vi "主动发送数据生成Condition(子VI).vi"(8 "数据发送协议":enum16{"2005-212协议", "2017-212协议"}(ring)=enum."2017-212协议", 9 "database":string, 10 "Label.Text":string, 11 "数值":i32) -> (2 "columns":string[](array[string])=["时间", "测量模式", "数据类型", "检测值", "单位", "数据标识"], 3 "CONDITION":string)   [LabVIEW 2016, in "数据传输系统.lvlib"]
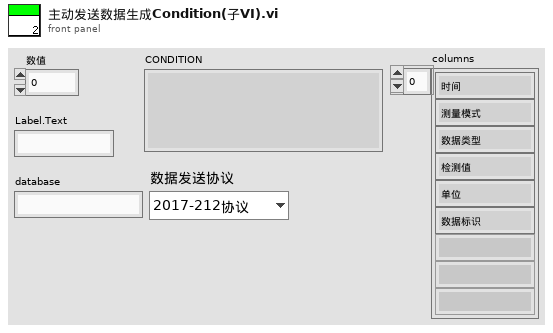
[diagram p1: front panel]
types:
  T1 = cluster{"time1":string, "time2":string, "time3":string, "time4":string, "time5":string, "time6":string, "time7":string, "time8":string, "time9":string, "time10":string, "time11":string, "time12":string, "time13":string, "time14":string, "time15":string, "time16":string, "time17":string, "time18":string, "time19":string, "time20":string, "time21":string, "time22":string, "time23":string, "time24":string, "time25":string, "time26":string, "time27":string, "time28":string, "time29":string, "time30":string, "time31":string}
  T2 = typedef "LVDateTimeRec.ctl" = cluster{"秒数的小数部分":dbl, "秒":i32, "分":i32, "时":i32, "日":i32, "月":i32, "年":i32, "天数（周）":i32, "天数（年）":i32, "DST":i32}
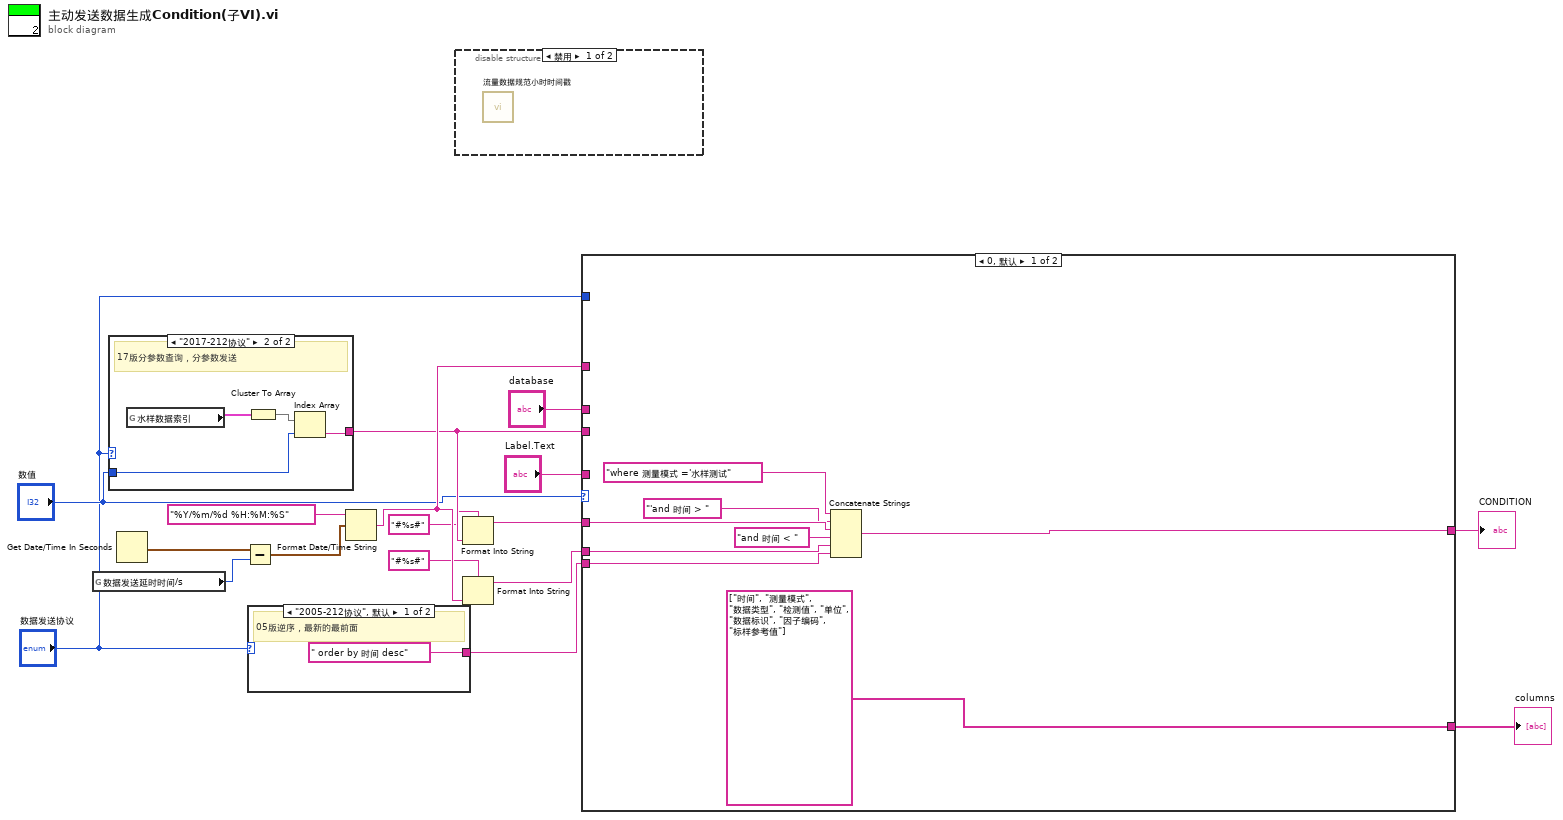
[diagram p0: block diagram]
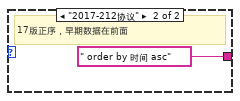
[diagram p3: hidden frame]
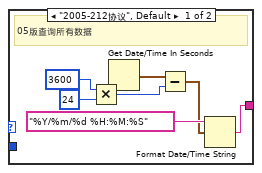
[diagram p4: hidden frame]
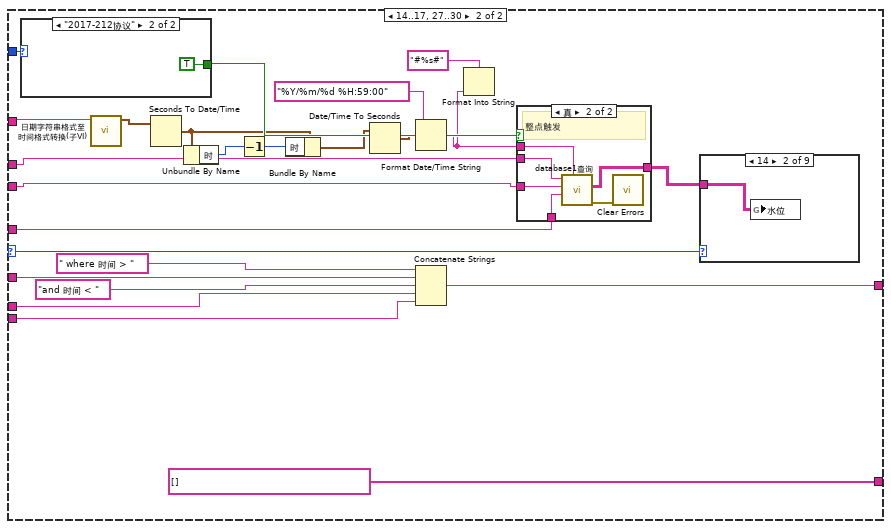
[diagram p5: hidden frame]
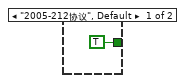
[diagram p6: hidden frame]
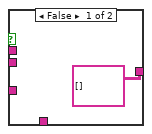
[diagram p7: hidden frame]
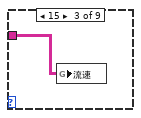
[diagram p9: hidden frame]
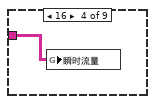
[diagram p10: hidden frame]
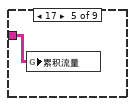
[diagram p11: hidden frame]
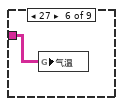
[diagram p12: hidden frame]
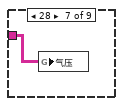
[diagram p13: hidden frame]
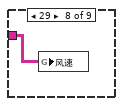
[diagram p14: hidden frame]
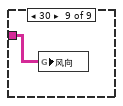
[diagram p15: hidden frame]
diagram:
  n1 = global read "断电保存全局.vi" "数据发送延时时间/s"() -> (w3:i32)
  n2 = case shown="\"2017-212协议\"" "数据发送协议" {
    tunnel: [w23 w25] -> w16
    tunnel: "数值" -> [_ w26]
    frame "2005-212协议", Default {
      # "05版查询所有数据"
      n3 = Multiply(x=3600, y=24) -> (x*y=w18:i32)
      n4 = Get Date/Time In Seconds() -> (seconds since 1Jan1904=w22:timestamp)
      n5 = Subtract(x=w22, y=w18) -> (x-y=w21:timestamp)
      n6 = Format Date/Time String(time format string (%c)="%Y/%m/%d %H:%M:%S" ("时间格式字符串(%c)"), seconds (now)=w21) -> (date/time string=w23:string)  [unwired: 1 in]
    }
    frame "2017-212协议" {
      # "17版分参数查询，分参数发送"
      n7 = global read "全局 水样时间.vi" "水样数据索引"() -> (w27:T1)
      n8 = Cluster To Array(cluster=w27) -> (array=w28:string[])
      n9 = Index Array(array=w28, index=w26) -> (element=w25:string)
    }
  }
  n10 = Get Date/Time In Seconds() -> (seconds since 1Jan1904=w2:timestamp)
  n11 = Subtract(x=w2, y=w3) -> (x-y=w1:timestamp)
  n12 = case shown="\"2005-212协议\", 默认" "数据发送协议" {
    tunnel: [" order by 时间 desc" ("字符串") " order by 时间 asc" ("字符串")] -> w6
    frame "2005-212协议", Default {
      # "05版逆序，最新的最前面"
    }
    frame "2017-212协议" {
      # "17版正序，早期数据在前面"
    }
  }
  n13 = Format Date/Time String(time format string (%c)="%Y/%m/%d %H:%M:%S" ("时间格式字符串(%c)"), seconds (now)=w1) -> (date/time string=w17:string)  [unwired: 1 in]
  n14 = disable-structure shown="禁用" {
    frame Disabled {
      n15 = call "流量数据规范小时时间戳.vi"() -> ()  [unwired: 11 in, 1 out]
    }
    frame Enabled {
    }
  }
  n16 = Format Into String(format string="#%s#" ("初始字符串"), w16) -> (resulting string=w10:string)  [unwired: 2 in, 1 out]
  n17 = Format Into String(format string="#%s#" ("初始字符串"), w17) -> (resulting string=w12:string)  [unwired: 2 in, 1 out]
  n18 = case shown="0, 默认" "数值" {
    selector: "数值" -> [_ w55]
    tunnel: w10 -> [w38 w59]
    tunnel: [w37 w60] -> w11
    tunnel: w12 -> [w35 w40]
    tunnel: "database" -> [_ w58]
    tunnel: "Label.Text" -> [_ w57]
    tunnel: w16 -> [_ w39]
    tunnel: w17 -> [_ w43]
    tunnel: w6 -> [w32 w54]
    tunnel: [string[] ["时间", "测量模式", "数据类型", "检测值", "单位", "数据标识", "因子编码", "标样参考值"] ("columns") string[] [] ("columns")] -> w5
    tunnel: "数据发送协议" -> [_ w51]
    frame 0, Default {
      n19 = Concatenate Strings("where 测量模式 ='水样测试" ("condition"), "'and 时间 > ", w38, "and 时间 < " ("字符串"), w35, w32) -> (w37:string)
    }
    frame 14..17, 27..30 {
      n20 = case shown="\"2017-212协议\"" w51 {
        tunnel: [TRUE TRUE] -> w53
        frame "2005-212协议", Default {
        }
        frame "2017-212协议" {
        }
      }
      n21 = call "日期字符串格式至时间格式转换(子VI).vi"("data[0]"=w43) -> ("time stamp"=w46:timestamp)  [unwired: 10 in]
      n22 = Seconds To Date/Time(time stamp (now)=w46) -> (date time rec=w48:T2)  [unwired: 1 in]
      n23 = Unbundle By Name(w48) -> ("时"=w49:i32)
      n24 = Decrement(x=w49) -> (x-1=w50:i32)
      n25 = Bundle By Name(cluster=w48, "时"=w50) -> (w47:T2)
      n26 = Date/Time To Seconds(2:w47) -> (0:w45:timestamp)  [unwired: 1 in]
      n27 = Format Date/Time String(time format string (%c)="%Y/%m/%d %H:59:00" ("时间格式字符串(%c)"), seconds (now)=w45) -> (date/time string=w41:string)  [unwired: 1 in]
      n28 = Concatenate Strings(" where 时间 > ", w59, "and 时间 < " ("字符串"), w40, w54) -> (w60:string)
      n29 = Format Into String(format string="#%s#" ("初始字符串"), w41) -> ()  [unwired: 2 in, 2 out]
      n30 = case shown="真" w53 {
        tunnel: w58 -> [_ w71]
        tunnel: w57 -> [_ w70]
        tunnel: [string[][] [] ("data") w69] -> w56
        tunnel: w41 -> [_ w68]
        tunnel: w39 -> [_ w66]
        frame False {
        }
        frame True {
          # "整点触发"
          n31 = call "database1查询.vi"("时间2"=w68, "table"=w70, "时间1"=w66, "database"=w71) -> ("error out"=w67:errorcluster, "data"=w69:string[][])  [unwired: 4 in, 1 out]
          n32 = call <vilib>:"Clear Errors.vi"("error in (no error)"=w67) -> ()  [unwired: 5 in, 2 out]
        }
      }
      n33 = case shown="14" w55 {
        tunnel: w56 -> [_ w72 w73 w74 w75 w76 w77 w78 w79]
        frame 0, Default {
        }
        frame 14 {
          n34 = global write "全局 所有参数.vi" "水位"(w72) -> ()
        }
        frame 15 {
          n35 = global write "全局 所有参数.vi" "流速"(w73) -> ()
        }
        frame 16 {
          n36 = global write "全局 所有参数.vi" "瞬时流量"(w74) -> ()
        }
        frame 17 {
          n37 = global write "全局 所有参数.vi" "累积流量"(w75) -> ()
        }
        frame 27 {
          n38 = global write "全局 所有参数.vi" "气温"(w76) -> ()
        }
        frame 28 {
          n39 = global write "全局 所有参数.vi" "气压"(w77) -> ()
        }
        frame 29 {
          n40 = global write "全局 所有参数.vi" "风速"(w78) -> ()
        }
        frame 30 {
          n41 = global write "全局 所有参数.vi" "风向"(w79) -> ()
        }
      }
    }
  }
  "CONDITION" <- w11
  "columns" <- w5
